vi "loadCTData.vi"() -> ()   [LabVIEW 2012]
uses:
  <vilib>/addons/database/Connection.llb/DB Tools Open Connec (Path).vi
  <vilib>/addons/database/Connection.llb/Conn Execute.vi
  <vilib>/addons/database/Recordset.llb/Rec Fetch Recordset Data (R).vi
  <vilib>/addons/database/Recordset.llb/Rec Destroy - Connection.vi
  <vilib>/addons/database/Recordset.llb/Rec Fetch Integer Data (R).vi
  <vilib>/addons/database/_DB Variant To Data/Database Variant To Data.xnode
  <vilib>/addons/database/NI_Database_API.lvlib
panel:
  out "data":string
  out "x = y?":bool
  out "concatenated string 3":string
  out "concatenated string 2":string
  out "concatenated string":string
  out "data 3":string
  out "error out":errorcluster
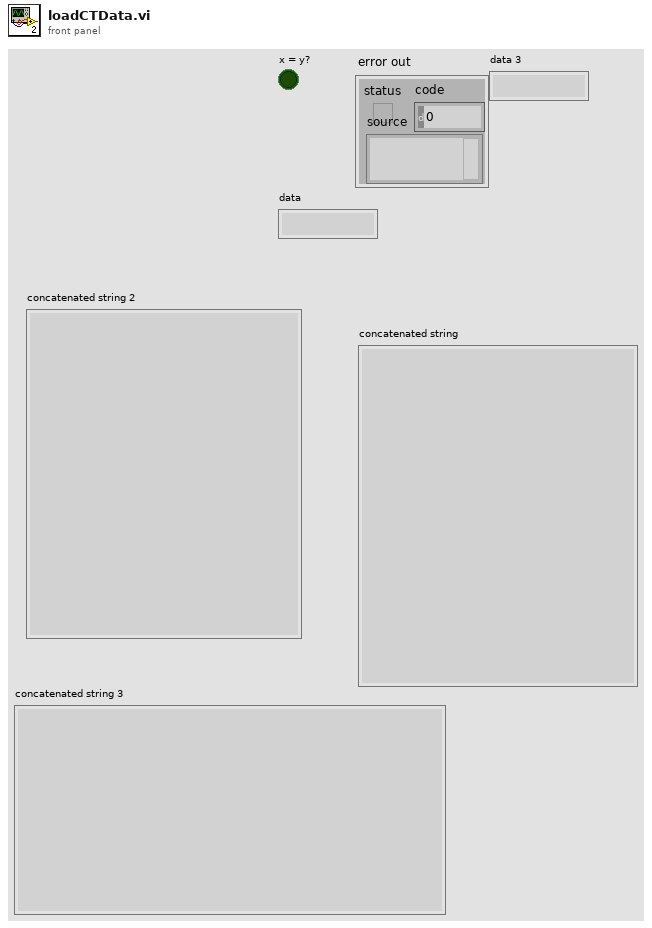
[diagram p1: front panel]
types:
  T1 = typedef "NI_Database_API.lvlib/Conn ObjectReference.ctl" = refnum<k1>
  T2 = typedef "NI_Database_API.lvlib/Rec ObjectReference.ctl" = refnum<k1>
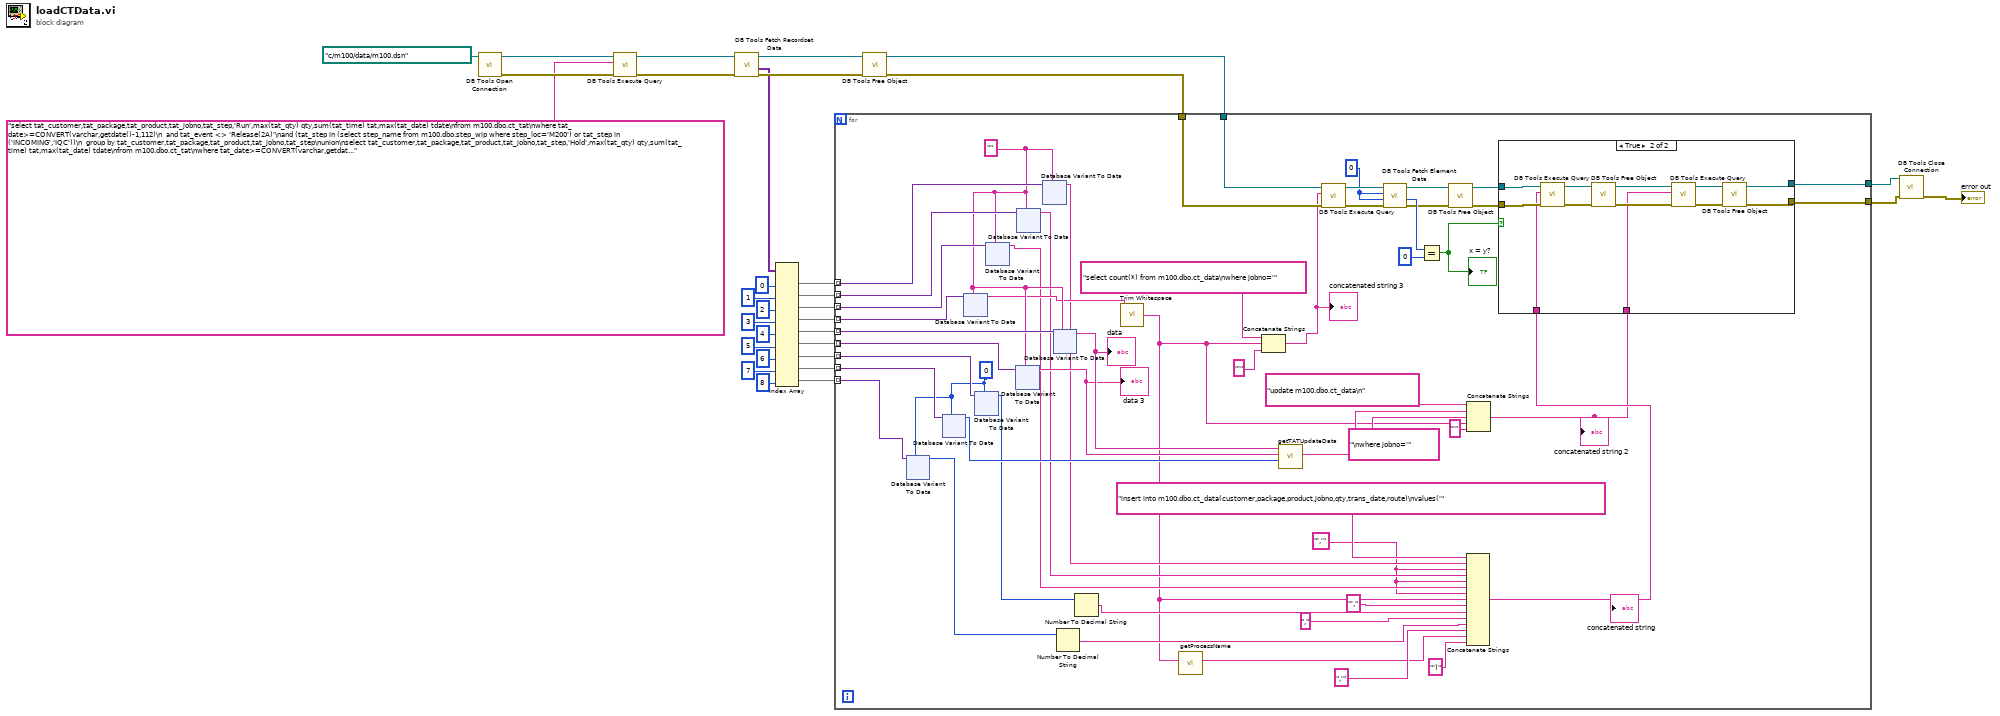
[diagram p0: block diagram]
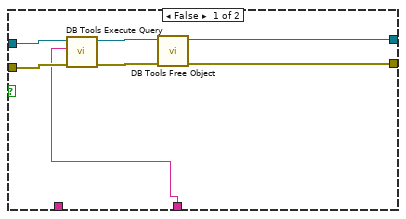
[diagram p2: hidden frame]
diagram:
  n1 = call-poly <vilib>:"DB Tools Open Connection.vi"("connection information"=path "c:/m100/data/m100.dsn") -> ("error out"=w29:errorcluster, "connection reference"=w32:T1)  [unwired: 7 in]
  n2 = call-poly <vilib>:"DB Tools Execute Query.vi"("error in (no error)"=w29, "SQL query"="select tat_customer,tat_package,tat_product,tat_jobno,tat_step,'Run',max(tat_qty) qty,sum(tat_time) tat,max(tat_date) tdate\nfrom m100.dbo.ct_tat\nwhere tat_date>=CONVERT(varchar,getdate()-1,112)\n  and tat_event <> 'Release(2A)'\nand (tat_step in (select step_name from m100.dbo.step_wip where step_loc='M200') or tat_step in ('INCOMING','IQC'))\n  group by tat_customer,tat_package,tat_product,tat_jobno,tat_step\nunion\nselect tat_customer,tat_package,tat_product,tat_jobno,tat_step,'Hold',max(tat_qty) qty,sum(tat_time) tat,max(tat_date) tdate\nfrom m100.dbo.ct_tat\nwhere tat_date>=CONVERT(varchar,getdate()-1,112)\n  and tat_event = 'Release(2A)'\nand (tat_step in (select step_name from m100.dbo.step_wip where step_loc='M200') or tat_step in ('INCOMING','IQC'))\n  group by tat_customer,tat_package,tat_product,tat_jobno,tat_step\n  order by tat_customer,tat_package,tat_product,tat_jobno,tat_step", "connection reference"=w32) -> ("error out"=w28:errorcluster, "recordset reference"=w31:T2)  [unwired: 5 in]
  n3 = call-poly <vilib>:"DB Tools Fetch Recordset Data.vi"("error in (no error)"=w28, "recordset reference"=w31) -> ("error out"=w27:errorcluster, "recordset data"=w23:variant[][], "recordset reference out"=w30:T2)  [unwired: 3 in]
  n4 = Index Array(array=w23, index (col) #1=0 ("disabled index (col)"), index (col) #2=1 ("index (col)"), index (col) #3=2 ("index (col)"), index (col) #4=3 ("index (col)"), index (col) #5=4 ("index (col)"), index (col) #6=5 ("index (col)"), index (col) #7=6 ("index (col)"), index (col) #8=7 ("index (col)"), index (col) #9=8 ("index (col)")) -> (element #1=w13:variant[], element #2=w12:variant[], element #3=w11:variant[], element #4=w10:variant[], element #5=w9:variant[], element #6=w8:variant[], element #7=w7:variant[], element #8=w6:variant[], element #9=w5:variant[])  [unwired: 9 in]
  n5 = call-poly <vilib>:"DB Tools Free Object.vi"("error in (no error)"=w27, "recordset reference"=w30) -> ("error out"=w3:errorcluster, "connection reference"=w4:T1)  [unwired: 8 in]
  n6 = for {
    tunnel: w13 -> [w85] mode=indexing
    tunnel: w12 -> [w84] mode=indexing
    tunnel: w11 -> [w83] mode=indexing
    tunnel: w10 -> [w77] mode=indexing
    tunnel: w9 -> [w82] mode=indexing
    tunnel: w8 -> [w81] mode=indexing
    tunnel: w7 -> [w80] mode=indexing
    tunnel: w6 -> [w79] mode=indexing
    tunnel: w5 -> [w78] mode=indexing
    tunnel: w4 -> [w74]
    tunnel: w3 -> [w73]
    tunnel: [w38] -> w2
    tunnel: [w37] -> w1
    w47 = "','" ("string")
    w67 = 0
    w75 = 0
    w76 = ""
    n7 = xnode "Database Variant To Data"("database variant"=w78, "type"=w75) -> ("data"=w42:i32)  [unwired: 1 in, 1 out]
    n8 = xnode "Database Variant To Data"("database variant"=w79, "type"=w75) -> ("data"=w58:i32)  [unwired: 1 in, 1 out]
    n9 = xnode "Database Variant To Data"("database variant"=w77, "type"=w76) -> ("data"=w61:string)  [unwired: 1 in, 1 out]
    n10 = xnode "Database Variant To Data"("database variant"=w80, "type"=w75) -> ("data"=w45:i32)  [unwired: 1 in, 1 out]
    n11 = xnode "Database Variant To Data"("database variant"=w83, "type"=w76) -> ("data"=w48:string)  [unwired: 1 in, 1 out]
    n12 = xnode "Database Variant To Data"("database variant"=w81, "type"=w76) -> ("data"=w59:string)  [unwired: 1 in, 1 out]
    "data 3" <- w59
    n13 = xnode "Database Variant To Data"("database variant"=w84, "type"=w76) -> ("data"=w49:string)  [unwired: 1 in, 1 out]
    n14 = xnode "Database Variant To Data"("database variant"=w85, "type"=w76) -> ("data"=w50:string)  [unwired: 1 in, 1 out]
    n15 = xnode "Database Variant To Data"("database variant"=w82, "type"=w76) -> ("data"=w60:string)  [unwired: 1 in, 1 out]
    "data" <- w60
    n16 = Number To Decimal String(number=w42) -> (decimal integer string=w41:string)  [unwired: 1 in]
    n17 = Number To Decimal String(number=w45) -> (decimal integer string=w44:string)  [unwired: 1 in]
    n18 = call <vilib>:"Trim Whitespace.vi"("string"=w61) -> ("trimmed string"=w36:string)  [unwired: 1 in]
    n19 = call "getProcessName.vi"("Lotno"=w36) -> ("ProcessName"=w33:string)  [unwired: 10 in]
    n20 = Concatenate Strings("select count(*) from m100.dbo.ct_data\nwhere jobno='" ("string"), w36, "'" ("string")) -> (w70:string)
    "concatenated string 3" <- w70
    n21 = call "getTATUpdateData.vi"("time"=w58, "Status"=w59, "step"=w60) -> ("updateData"=w57:string)  [unwired: 8 in]
    n22 = call-poly <vilib>:"DB Tools Execute Query.vi"("error in (no error)"=w73, "SQL query"=w70, "connection reference"=w74) -> ("error out"=w68:errorcluster, "recordset reference"=w69:T2)  [unwired: 5 in]
    n23 = call-poly <vilib>:"DB Tools Fetch Element Data.vi"("error in (no error)"=w68, "type"=w67, "column index"=w67, "recordset reference"=w69) -> ("error out"=w63:errorcluster, "data"=w66:i32, "recordset reference out"=w64:T2)  [unwired: 3 in]
    n24 = Equal?(x=w66, y=0) -> (x = y?=w51:bool)
    "x = y?" <- w51
    n25 = call-poly <vilib>:"DB Tools Free Object.vi"("error in (no error)"=w63, "recordset reference"=w64) -> ("error out"=w53:errorcluster, "connection reference"=w54:T1)  [unwired: 8 in]
    n26 = Concatenate Strings("insert into m100.dbo.ct_data(customer,package,product,jobno,qty,trans_date,route)\nvalues('" ("string"), w50, w47, w49, w47, w48, w47, w36, "'," ("string"), w44, "," ("string"), w41, ",'" ("string"), w33, "')" ("string")) -> (w40:string)
    "concatenated string" <- w40
    n27 = Concatenate Strings("update m100.dbo.ct_data\n" ("string"), w57, "\nwhere jobno='" ("string"), w36, "'" ("string")) -> (w39:string)
    "concatenated string 2" <- w39
    n28 = case shown="True" w51 {
      tunnel: w54 -> [w90 w102]
      tunnel: w53 -> [w89 w101]
      tunnel: w40 -> [_ w96]
      tunnel: w39 -> [w88 w95]
      tunnel: [w87 w94] -> w38
      tunnel: [w86 w93] -> w37
      frame False {
        n29 = call-poly <vilib>:"DB Tools Execute Query.vi"("error in (no error)"=w89, "SQL query"=w88, "connection reference"=w90) -> ("error out"=w92:errorcluster, "recordset reference"=w91:T2)  [unwired: 5 in]
        n30 = call-poly <vilib>:"DB Tools Free Object.vi"("error in (no error)"=w92, "recordset reference"=w91) -> ("error out"=w86:errorcluster, "connection reference"=w87:T1)  [unwired: 8 in]
      }
      frame True {
        n31 = call-poly <vilib>:"DB Tools Execute Query.vi"("error in (no error)"=w101, "SQL query"=w96, "connection reference"=w102) -> ("error out"=w104:errorcluster, "recordset reference"=w103:T2)  [unwired: 5 in]
        n32 = call-poly <vilib>:"DB Tools Free Object.vi"("error in (no error)"=w104, "recordset reference"=w103) -> ("error out"=w97:errorcluster, "connection reference"=w98:T1)  [unwired: 8 in]
        n33 = call-poly <vilib>:"DB Tools Execute Query.vi"("error in (no error)"=w97, "SQL query"=w95, "connection reference"=w98) -> ("error out"=w100:errorcluster, "recordset reference"=w99:T2)  [unwired: 5 in]
        n34 = call-poly <vilib>:"DB Tools Free Object.vi"("error in (no error)"=w100, "recordset reference"=w99) -> ("error out"=w93:errorcluster, "connection reference"=w94:T1)  [unwired: 8 in]
      }
    }
  }
  n35 = call <vilib>:"DB Tools Close Connection.vi"("error in (no error)"=w1, "connection reference"=w2) -> ("error out"=→"error out":errorcluster)  [unwired: 5 in]
